vi "P-612 Control.vi"(0 "P-612 Notifier":refnum<notifier>, 5 "Stage Actions":T1={"Action"=enum."Get Position", "Axis"=[], "Setpoint"=[], "Velocity"=0.5, "Cmd Recvd?"=FALSE, "Position"=[], "Status"=enum."Error", "Misc"=variant} {"Velocity" min=0.0 max=1.0 step=0.01}, 11 "VISA In":refnum<visa-resource-name>, 13 "Axis Names":string[](array[string])) -> (4 "P-612 Notifier (Dup)":refnum<notifier>)   [LabVIEW 2016]
uses:
  Stages Controls/Stage Notifier Element.ctl
  Stages Controls/Stage Actions.ctl
  Stages Controls/Stage Status.ctl
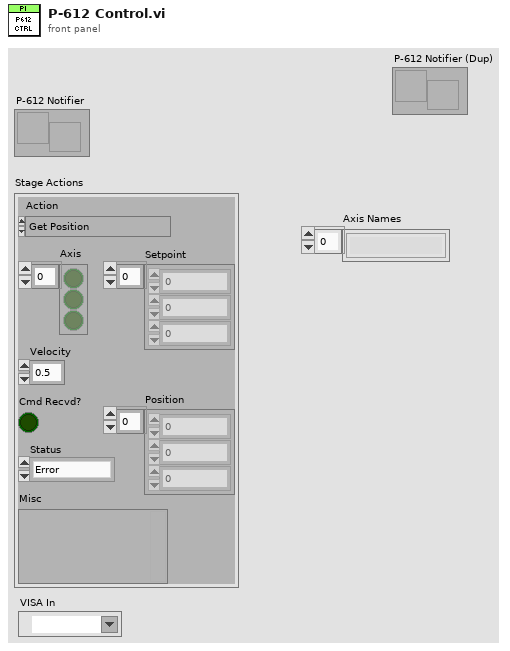
[diagram p1: front panel]
types:
  T1 = typedef "Stage Notifier Element.ctl" = cluster{"Action":T2, "Axis":bool[], "Setpoint":dbl[], "Velocity":dbl, "Cmd Recvd?":bool, "Position":dbl[], "Status":T3, "Misc":variant}
  T2 = typedef "Stage Actions.ctl" = enum16{"Get Position", "MVR", "MOVE", "HALT", "ONTARGET", "ERROR", "REFERENCE", "INIT", "VELOCITY", "STATUS", "EXIT", "HOME", "ZEROPOS", "NANOPOS", "ANALOG", "QUIT"}
  T3 = typedef "Stage Status.ctl" = enum16{"Error", "Abort", "Busy", "On Target"}
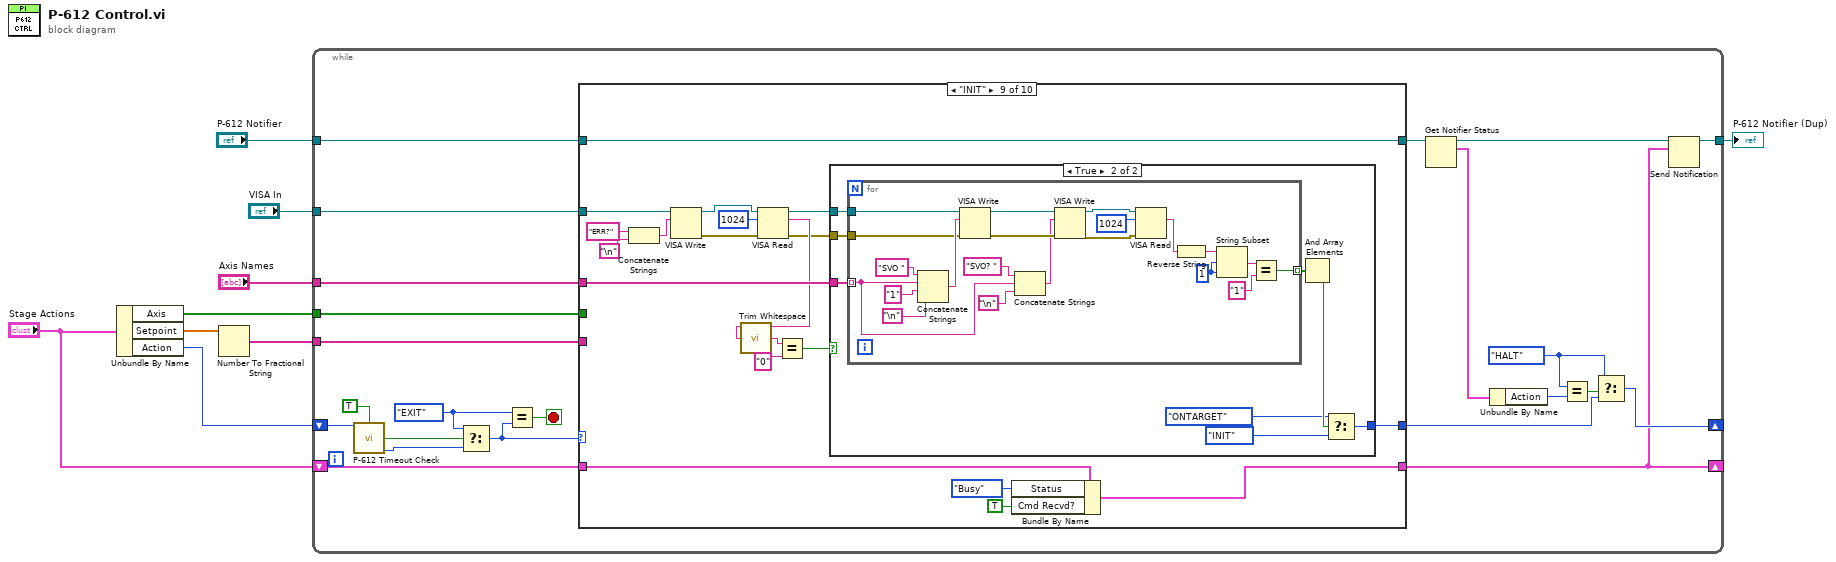
[diagram p0: block diagram]
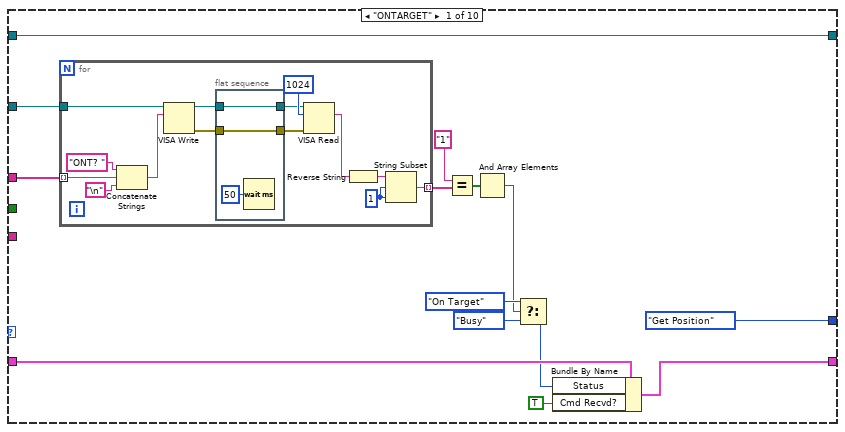
[diagram p2: hidden frame]
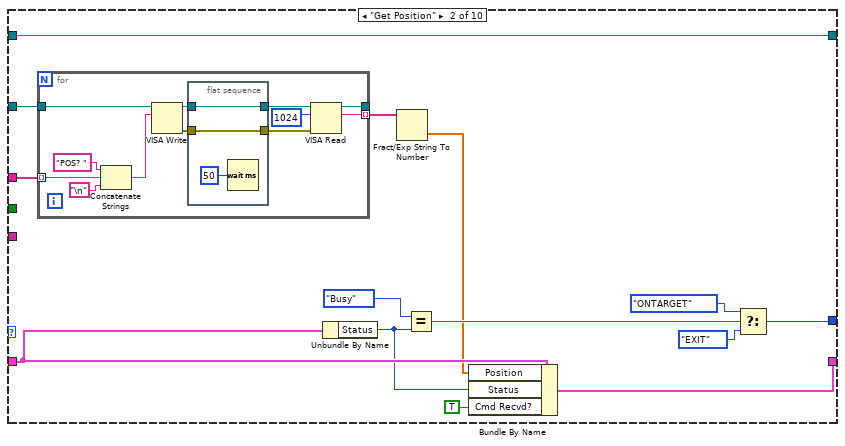
[diagram p3: hidden frame]
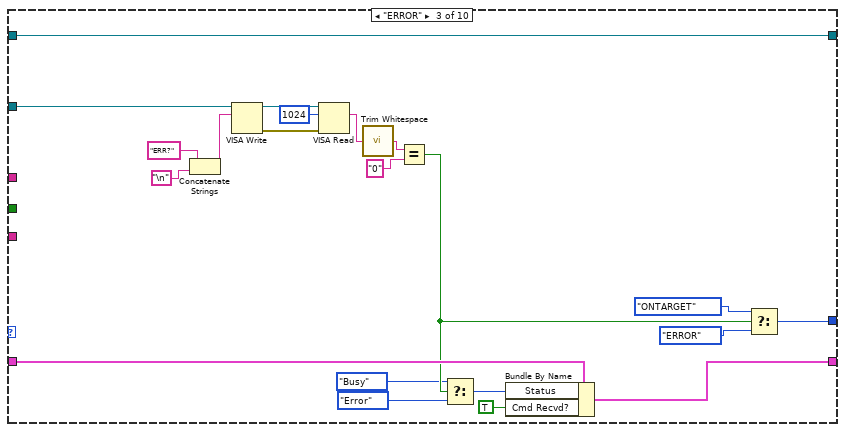
[diagram p4: hidden frame]
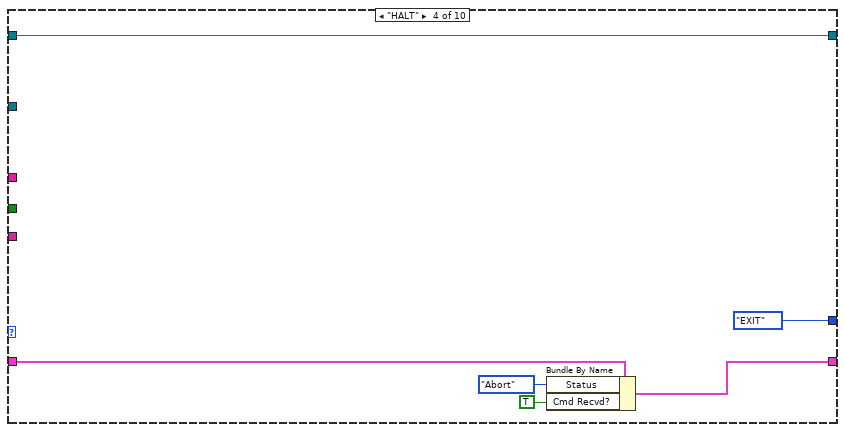
[diagram p5: hidden frame]
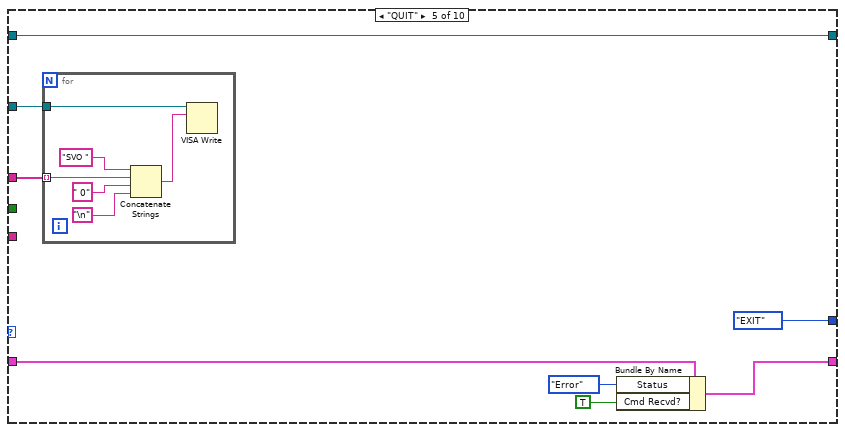
[diagram p6: hidden frame]
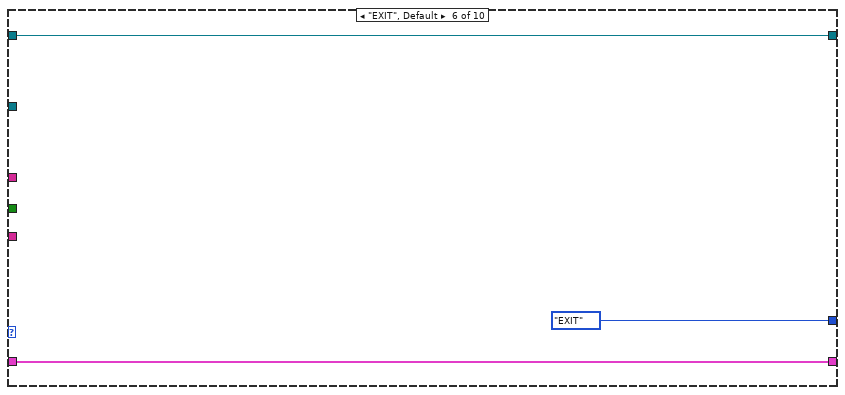
[diagram p7: hidden frame]
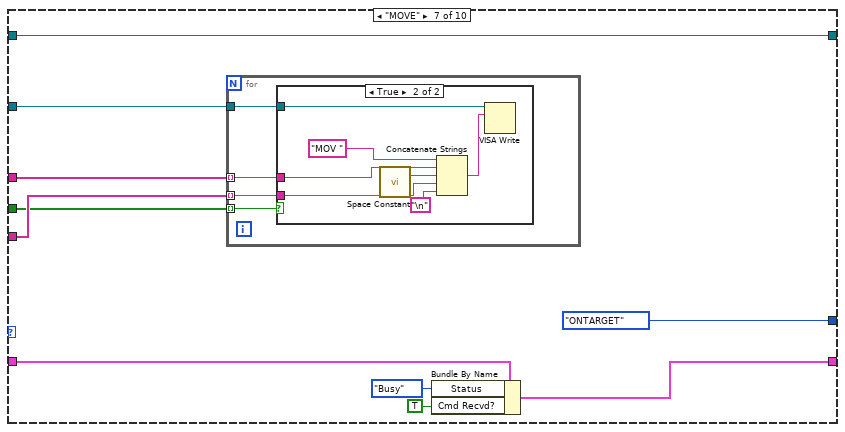
[diagram p8: hidden frame]
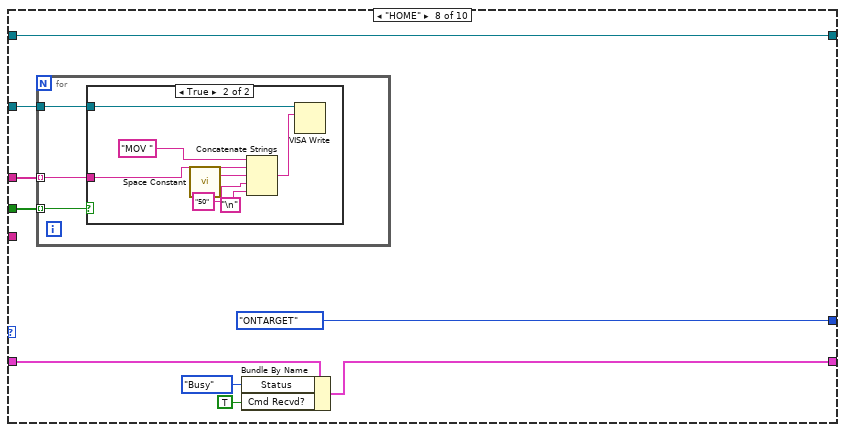
[diagram p10: hidden frame]
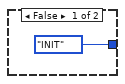
[diagram p12: hidden frame]
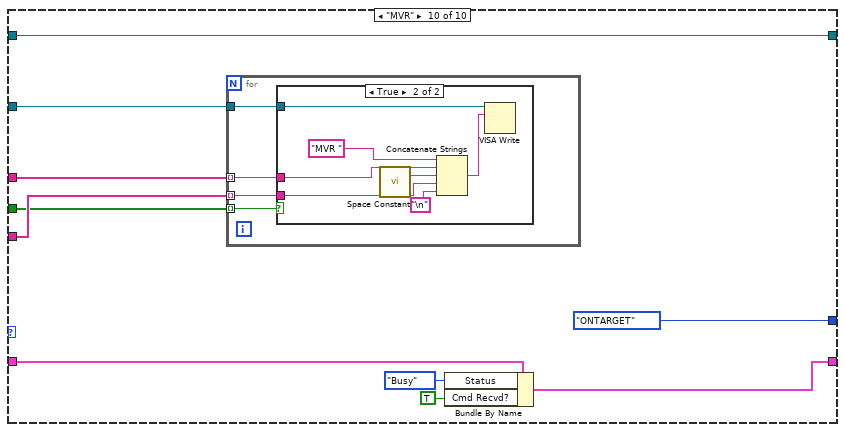
[diagram p13: hidden frame]
diagram:
  n1 = Unbundle By Name("Stage Actions") -> ("Axis"=w8:bool[], "Setpoint"=w7:dbl[], "Action"=w6:T2)
  n2 = Number To Fractional String(number=w7) -> (F-format string=w9:string[])  [unwired: 3 in]
  n3 = while {
    tunnel: "Axis Names" -> [w32]
    shift-right: [w27] -> _
    shift-left: w6 -> [w24]
    tunnel: w8 -> [w30]
    tunnel: w9 -> [w31]
    shift-right: [w26] -> _
    shift-left: "Stage Actions" -> [w29]
    tunnel: "P-612 Notifier" -> [w18]
    tunnel: "VISA In" -> [w17]
    tunnel: [w10] -> w2
    stop <- w19 stop-if-true
    w13 = Stage_Actions."HALT" ("Action")
    w23 = Stage_Actions."EXIT" ("t")
    n4 = call "P-612 Timeout Check.vi"("Action"=w24, "User Input?"=TRUE) -> ("Timeout?"=w22:bool, "Action (Dup)"=w21:T2)  [unwired: 12 in]
    n5 = Select(t=w23, s=w22, f=w21) -> (s? t:f=w20:T2)
    n6 = Equal?(x=w23, y=w20) -> (x = y?=w19:bool)
    n7 = case shown="\"INIT\"" w20 {
      tunnel: w32 -> [w46 w77 _ _ w126 _ w146 w166 w196 w236]
      tunnel: w31 -> [_ _ _ _ _ _ w145 _ _ w235]
      tunnel: w30 -> [_ _ _ _ _ _ w144 w165 _ w234]
      tunnel: [Stage_Actions."Get Position" ("y") w75 w102 Stage_Actions."EXIT" ("y") Stage_Actions."EXIT" ("y") Stage_Actions."EXIT" ("y") Stage_Actions."ONTARGET" ("y") Stage_Actions."ONTARGET" ("y") w191 Stage_Actions."ONTARGET" ("y")] -> w28
      tunnel: w29 -> [w40 w73 w97 w115 w124 w136 w141 w162 w193 w231]
      tunnel: [w41 w70 w98 w116 w123 w136 w140 w161 w192 w230] -> w26
      tunnel: w18 -> [w34 w64 w93 w114 w120 w134 w137 w159 w177 w227]
      tunnel: [w34 w64 w93 w114 w120 w134 w137 w159 w177 w227] -> w11
      tunnel: w17 -> [w33 w65 w94 _ w121 _ w138 w158 w178 w228]
      frame "ONTARGET" {
        n8 = for {
          tunnel: w46 -> [w60] mode=indexing
          tunnel: [w59] -> w45 mode=indexing
          tunnel: w33 -> [w47]
          w54 = 1 ("length (rest)")
          n9 = Concatenate Strings("ONT? " ("string"), w60, "\n") -> (w53:string)
          n10 = VISA Write(VISA resource name=w47, write buffer=w53) -> (VISA resource name out=w50:refnum<visa-resource-name>, error out=w48:errorcluster)  [unwired: 1 in, 1 out]
          n11 = flat-sequence {
            tunnel: [w63] -> w51
            tunnel: w50 -> [w63]
            tunnel: [w62] -> w49
            tunnel: w48 -> [w62]
            frame #0 {
              n12 = Wait (ms)(milliseconds to wait=u32 50) -> ()  [unwired: 1 out]
            }
          }
          n13 = VISA Read(VISA resource name=w51, byte count=u32 1024, error in (no error)=w49) -> (read buffer=w52:string)  [unwired: 3 out]
          n14 = Reverse String(1:w52) -> (0:w55:string)
          n15 = String Subset(string=w55, offset (0)=w54, length (rest)=w54) -> (substring=w59:string)
        }
        n16 = Equal?(x="1", y=w45) -> (x = y?=w43:bool[])
        n17 = And Array Elements(Boolean array=w43) -> (logical AND=w37:bool)
        n18 = Select(t=Stage_Status."On Target" ("Status"), s=w37, f=Stage_Status."Busy" ("Status")) -> (s? t:f=w36:T3)
        n19 = Bundle By Name(cluster=w40, "Status"=w36, "Cmd Recvd?"=TRUE) -> (w41:T1)
      }
      frame "Get Position" {
        n20 = for {
          tunnel: w77 -> [w89] mode=indexing
          tunnel: [w84] -> w76 mode=indexing
          tunnel: [w79] -> _
          tunnel: w65 -> [w78]
          n21 = Concatenate Strings("POS? " ("string"), w89, "\n") -> (w85:string)
          n22 = VISA Write(VISA resource name=w78, write buffer=w85) -> (VISA resource name out=w82:refnum<visa-resource-name>, error out=w80:errorcluster)  [unwired: 1 in, 1 out]
          n23 = flat-sequence {
            tunnel: [w92] -> w83
            tunnel: w82 -> [w92]
            tunnel: [w91] -> w81
            tunnel: w80 -> [w91]
            frame #0 {
              n24 = Wait (ms)(milliseconds to wait=u32 50) -> ()  [unwired: 1 out]
            }
          }
          n25 = VISA Read(VISA resource name=w83, byte count=u32 1024, error in (no error)=w81) -> (VISA resource name out=w79:refnum<visa-resource-name>, read buffer=w84:string)  [unwired: 2 out]
        }
        n26 = Unbundle By Name(w73) -> ("Status"=w68:T3)
        n27 = Fract/Exp String To Number(string=w76) -> (number=w69:dbl[])  [unwired: 3 in, 1 out]
        n28 = Equal?(x=Stage_Status."Busy", y=w68) -> (x = y?=w71:bool)
        n29 = Bundle By Name(cluster=w73, "Position"=w69, "Status"=w68, "Cmd Recvd?"=TRUE) -> (w70:T1)
        n30 = Select(t=Stage_Actions."ONTARGET" ("y"), s=w71, f=Stage_Actions."EXIT" ("y")) -> (s? t:f=w75:T2)
      }
      frame "ERROR" {
        n31 = Concatenate Strings("ERR?" ("string"), "\n") -> (w106:string)
        n32 = VISA Write(VISA resource name=w94, write buffer=w106) -> (VISA resource name out=w105:refnum<visa-resource-name>, error out=w110:errorcluster)  [unwired: 1 in, 1 out]
        n33 = VISA Read(VISA resource name=w105, byte count=u32 1024, error in (no error)=w110) -> (read buffer=w111:string)  [unwired: 3 out]
        n34 = call <vilib>:"Trim Whitespace.vi"("string"=w111) -> ("trimmed string"=w113:string)  [unwired: 1 in]
        n35 = Equal?(x=w113, y="0") -> (x = y?=w96:bool)
        n36 = Select(t=Stage_Status."Busy" ("Status"), s=w96, f=Stage_Status."Error" ("Status")) -> (s? t:f=w100:T3)
        n37 = Bundle By Name(cluster=w97, "Status"=w100, "Cmd Recvd?"=TRUE) -> (w98:T1)
        n38 = Select(t=Stage_Actions."ONTARGET" ("Action"), s=w96, f=Stage_Actions."ERROR") -> (s? t:f=w102:T2)
      }
      frame "HALT" {
        n39 = Bundle By Name(cluster=w115, "Status"=Stage_Status."Abort", "Cmd Recvd?"=TRUE) -> (w116:T1)
      }
      frame "QUIT" {
        n40 = for {
          tunnel: w126 -> [w130] mode=indexing
          tunnel: w121 -> [w128]
          n41 = Concatenate Strings("SVO " ("write buffer"), w130, " 0" ("string"), "\n") -> (w129:string)
          n42 = VISA Write(VISA resource name=w128, write buffer=w129) -> ()  [unwired: 1 in, 3 out]
        }
        n43 = Bundle By Name(cluster=w124, "Status"=Stage_Status."Error", "Cmd Recvd?"=TRUE) -> (w123:T1)
      }
      frame "EXIT", Default {
      }
      frame "MOVE" {
        n44 = for {
          tunnel: w146 -> [w150] mode=indexing
          tunnel: w145 -> [w149] mode=indexing
          tunnel: w144 -> [w148] mode=indexing
          tunnel: w138 -> [w147]
          n45 = case shown="True" w148 {
            tunnel: w150 -> [_ w155]
            tunnel: w149 -> [_ w152]
            tunnel: w147 -> [_ w151]
            frame False {
            }
            frame True {
              n46 = call <vilib>:"Space Constant.vi"() -> ("String"=w153:string)
              n47 = Concatenate Strings("MOV ", w155, w153, w152, "\n") -> (w157:string)
              n48 = VISA Write(VISA resource name=w151, write buffer=w157) -> ()  [unwired: 1 in, 3 out]
            }
          }
        }
        n49 = Bundle By Name(cluster=w141, "Status"=Stage_Status."Busy", "Cmd Recvd?"=TRUE) -> (w140:T1)
      }
      frame "HOME" {
        n50 = for {
          tunnel: w166 -> [w169] mode=indexing
          tunnel: w165 -> [w168] mode=indexing
          tunnel: w158 -> [w167]
          n51 = case shown="True" w168 {
            tunnel: w169 -> [_ w174]
            tunnel: w167 -> [_ w170]
            frame False {
            }
            frame True {
              n52 = call <vilib>:"Space Constant.vi"() -> ("String"=w172:string)
              n53 = Concatenate Strings("MOV ", w174, w172, "50" ("string"), "\n") -> (w176:string)
              n54 = VISA Write(VISA resource name=w170, write buffer=w176) -> ()  [unwired: 1 in, 3 out]
            }
          }
        }
        n55 = Bundle By Name(cluster=w162, "Status"=Stage_Status."Busy", "Cmd Recvd?"=TRUE) -> (w161:T1)
      }
      frame "INIT" {
        n56 = Concatenate Strings("ERR?" ("string"), "\n") -> (w188:string)
        n57 = VISA Write(VISA resource name=w178, write buffer=w188) -> (VISA resource name out=w183:refnum<visa-resource-name>, error out=w181:errorcluster)  [unwired: 1 in, 1 out]
        n58 = VISA Read(VISA resource name=w183, byte count=u32 1024, error in (no error)=w181) -> (VISA resource name out=w182:refnum<visa-resource-name>, read buffer=w185:string, error out=w180:errorcluster)  [unwired: 1 out]
        n59 = call <vilib>:"Trim Whitespace.vi"("string"=w185) -> ("trimmed string"=w187:string)  [unwired: 1 in]
        n60 = Equal?(x=w187, y="0") -> (x = y?=w179:bool)
        n61 = case shown="True" w179 {
          tunnel: w196 -> [_ w205]
          tunnel: [Stage_Actions."INIT" ("y") w201] -> w191
          tunnel: w182 -> [_ w198]
          tunnel: w180 -> [_ w199]
          frame False {
          }
          frame True {
            n62 = for {
              tunnel: w205 -> [w213] mode=indexing
              tunnel: [w210] -> w204 mode=indexing
              tunnel: w199 -> [w209]
              tunnel: w198 -> [w206]
              w222 = 1 ("length (rest)")
              n63 = Concatenate Strings("SVO " ("string"), w213, "1" ("string"), "\n") -> (w214:string)
              n64 = VISA Write(VISA resource name=w206, write buffer=w214, error in (no error)=w209) -> (VISA resource name out=w208:refnum<visa-resource-name>, error out=w226:errorcluster)  [unwired: 1 out]
              n65 = Concatenate Strings("SVO? " ("string"), w213, "\n") -> (w212:string)
              n66 = VISA Write(VISA resource name=w208, write buffer=w212, error in (no error)=w226) -> (VISA resource name out=w207:refnum<visa-resource-name>, error out=w225:errorcluster)  [unwired: 1 out]
              n67 = VISA Read(VISA resource name=w207, byte count=u32 1024, error in (no error)=w225) -> (read buffer=w223:string)  [unwired: 3 out]
              n68 = Reverse String(1:w223) -> (0:w221:string)
              n69 = String Subset(string=w221, offset (0)=w222, length (rest)=w222) -> (substring=w224:string)
              n70 = Equal?(x=w224, y="1") -> (x = y?=w210:bool)
            }
            n71 = And Array Elements(Boolean array=w204) -> (logical AND=w203:bool)
            n72 = Select(t=Stage_Actions."ONTARGET" ("y"), s=w203, f=Stage_Actions."INIT" ("y")) -> (s? t:f=w201:T2)
          }
        }
        n73 = Bundle By Name(cluster=w193, "Status"=Stage_Status."Busy", "Cmd Recvd?"=TRUE) -> (w192:T1)
      }
      frame "MVR" {
        n74 = for {
          tunnel: w236 -> [w240] mode=indexing
          tunnel: w235 -> [w239] mode=indexing
          tunnel: w234 -> [w238] mode=indexing
          tunnel: w228 -> [w237]
          n75 = case shown="True" w238 {
            tunnel: w240 -> [_ w245]
            tunnel: w239 -> [_ w242]
            tunnel: w237 -> [_ w241]
            frame False {
            }
            frame True {
              n76 = call <vilib>:"Space Constant.vi"() -> ("String"=w243:string)
              n77 = Concatenate Strings("MVR ", w245, w243, w242, "\n") -> (w247:string)
              n78 = VISA Write(VISA resource name=w241, write buffer=w247) -> ()  [unwired: 1 in, 3 out]
            }
          }
        }
        n79 = Bundle By Name(cluster=w231, "Status"=Stage_Status."Busy", "Cmd Recvd?"=TRUE) -> (w230:T1)
      }
    }
    n80 = Get Notifier Status(notifier=w11) -> (notifier out=w16:refnum<notifier>, current notification=w12:T1)  [unwired: 1 in, 3 out]
    n81 = Unbundle By Name(w12) -> ("Action"=w14:T2)
    n82 = Equal?(x=w13, y=w14) -> (x = y?=w15:bool)
    n83 = Select(t=w13, s=w15, f=w28) -> (s? t:f=w27:T2)
    n84 = Send Notification(notification=w26, notifier=w16) -> (notifier out=w10:refnum<notifier>)  [unwired: 1 in, 1 out]
  }
  "P-612 Notifier (Dup)" <- w2
